vi "HFRR ADV v12.vi"() -> ()   [LabVIEW 2025] (continued)
                frame 88 {
                  n3635 = local write "S 90"(w4921) -> ()
                }
                frame 89 {
                  n3636 = local write "S 91"(w4922) -> ()
                }
                frame 90 {
                  n3637 = local write "S 92"(w4923) -> ()
                }
                frame 91 {
                  n3638 = local write "S 93"(w4924) -> ()
                }
                frame 92 {
                  n3639 = local write "S 94"(w4925) -> ()
                }
                frame 93 {
                  n3640 = local write "S 95"(w4926) -> ()
                }
                frame 94 {
                  n3641 = local write "S 96"(w4927) -> ()
                }
                frame 95 {
                  n3642 = local write "S 97"(w4928) -> ()
                }
                frame 96 {
                  n3643 = local write "S 98"(w4929) -> ()
                }
                frame 97 {
                  n3644 = local write "S 99"(w4930) -> ()
                }
                frame 98 {
                  n3645 = local write "S 100"(w4931) -> ()
                }
                frame 99 {
                  n3646 = local write "S 101"(w4932) -> ()
                }
                frame 100 {
                  n3647 = local write "S 102"(w4933) -> ()
                }
                frame 101 {
                  n3648 = local write "S 103"(w4934) -> ()
                }
                frame 102 {
                  n3649 = local write "S 104"(w4935) -> ()
                }
                frame 103 {
                  n3650 = local write "S 105"(w4936) -> ()
                }
                frame 104 {
                  n3651 = local write "S 106"(w4937) -> ()
                }
                frame 105 {
                }
                frame 106 {
                  n3652 = property on="OK Button 17" class="Bool (strict)"("Boolean Text.Text"=w4938) -> ()  [unwired: 2 in, 2 out]
                }
                frame 107 {
                  n3653 = property on="OK Button 16" class="Bool (strict)"("Boolean Text.Text"=w4939) -> ()  [unwired: 2 in, 2 out]
                }
                frame 108 {
                  n3654 = property on="TITTLE" class="Str"("Caption.Text"=w4940) -> ()  [unwired: 2 in, 2 out]
                }
                frame 109 {
                  "String 30" <- w4941
                }
                frame 110 {
                  n3655 = property on="Test Date" class="Str"("Caption.Text"=w4942) -> ()  [unwired: 2 in, 2 out]
                  "String 31" <- w4942
                }
                frame 111 {
                  n3656 = property on="Sample ID" class="Str"("Caption.Text"=w4943) -> ()  [unwired: 2 in, 2 out]
                  "String 32" <- w4943
                }
                frame 112 {
                  n3657 = property on="Tested by" class="Str"("Caption.Text"=w4944) -> ()  [unwired: 2 in, 2 out]
                  "String 33" <- w4944
                }
                frame 113 {
                  n3658 = property on="System Configured Printers 2" class="Arr (strict)"("Caption.Text"=w4945) -> ()  [unwired: 2 in, 2 out]
                }
                frame 114 {
                  n3659 = property on="Selected Printer" class="Str"("Caption.Text"=w4946) -> ()  [unwired: 2 in, 2 out]
                }
                frame 115 {
                  n3660 = property on="Select Printer 3" class="DigNum (strict)"("Caption.Text"=w4947) -> ()  [unwired: 2 in, 2 out]
                }
                frame 116 {
                  n3661 = property on="Print" class="Bool (strict)"("Boolean Text.Text"=w4948) -> ()  [unwired: 2 in, 2 out]
                }
                frame 117 {
                  "String 41" <- w4949
                }
                frame 118 {
                  n3662 = property on="tested by" class="Str"("Caption.Text"=w4950) -> ()  [unwired: 2 in, 2 out]
                }
                frame 119 {
                }
                frame 120 {
                  n3663 = property on="Export" class="Bool (strict)"("Boolean Text.Text"=w4951) -> ()  [unwired: 2 in, 2 out]
                }
                frame 121 {
                  n3664 = property on="TEMP INTERCEPT:" class="DigNum (strict)"("Caption.Text"=w4952) -> ()  [unwired: 2 in, 2 out]
                }
                frame 122 {
                  n3665 = property on="AIR TEMP INTERCEPT:" class="DigNum (strict)"("Caption.Text"=w4953) -> ()  [unwired: 2 in, 2 out]
                }
                frame 123 {
                  n3666 = property on="Select File Type" class="Enum (strict)"("Caption.Text"=w4954) -> ()  [unwired: 2 in, 2 out]
                }
                frame 124 {
                  n3667 = property on="s.NO" class="Str"("Caption.Text"=w4955) -> ()  [unwired: 2 in, 2 out]
                  "String 45" <- w4955
                }
                frame 125 {
                  n3668 = property on="trip1 8" class="Bool (strict)"("Boolean Text.Text"=w4956) -> ()  [unwired: 2 in, 2 out]
                }
                frame 126, Default {
                }
              }
            }
          }
          frame #1 {
            w4964 = TRUE ("Visible")
            n3669 = local read "S 91"() -> (w4981:string)
            n3670 = local read "S 90"() -> (w4980:string)
            n3671 = local read "S 88"() -> (w4979:string)
            n3672 = property on="Threshold" class="DigNum (strict)"("Caption.Text"=w4981) -> ()  [unwired: 2 in, 2 out]
            n3673 = property on="File Path" class="Path"("Caption.Text"=w4980) -> ()  [unwired: 2 in, 2 out]
            n3674 = property on="SrvM CP" class="Bool (strict)"("Boolean Text.Text"=w4979) -> ()  [unwired: 2 in, 2 out]
            n3675 = local read "S 71"() -> (w4974:string)
            n3676 = local read "S 86"() -> (w4976:string)
            n3677 = local read "S 85"() -> (w4977:string)
            n3678 = local read "S 87"() -> (w4975:string)
            n3679 = local read "S 84"() -> (w4978:string)
            n3680 = local read "S 103"() -> (w4963:string)
            n3681 = local read "S 104"() -> (w4962:string)
            n3682 = property on="ENTER THE NEW PASSWORD" class="Str"("Caption.Text"=w4975) -> ()  [unwired: 2 in, 2 out]
            n3683 = property on="Password" class="Str"("Caption.Text"=w4977) -> ()  [unwired: 2 in, 2 out]
            n3684 = property on="ENTER CURRENT PASSWORD" class="Str"("Caption.Text"=w4976) -> ()  [unwired: 2 in, 2 out]
            n3685 = property on="EDIT" class="Bool (strict)"("Boolean Text.Text"=w4974) -> ()  [unwired: 2 in, 2 out]
            n3686 = property on="SAVE" class="Bool (strict)"("Boolean Text.Text"=w4978) -> ()  [unwired: 2 in, 2 out]
            n3687 = Build Array(w4963, w4962) -> (w4961:string[])
            n3688 = property on="Heater Button" class="Bool (strict)"("Strings [4]"=w4961) -> ()  [unwired: 2 in, 2 out]
            n3689 = property on="CH-HUMIDITY WET" class="DigNum (strict)"("Caption.Size to Text?"=w4964) -> ()  [unwired: 2 in, 2 out]
            n3690 = property on="CH-HUMIDITY DRY" class="DigNum (strict)"("Caption.Size to Text?"=w4964) -> ()  [unwired: 2 in, 2 out]
            n3691 = property on="CH-POWER -" class="DigNum (strict)"("Caption.Size to Text?"=w4964) -> ()  [unwired: 2 in, 2 out]
            n3692 = property on="CH-HEATER" class="DigNum (strict)"("Caption.Size to Text?"=w4964) -> ()  [unwired: 2 in, 2 out]
            n3693 = property on="CH-POWER +" class="DigNum (strict)"("Caption.Size to Text?"=w4964) -> ()  [unwired: 2 in, 2 out]
            n3694 = local read "S 92"() -> (w4973:string)
            n3695 = local read "S 93"() -> (w4972:string)
            n3696 = local read "S 105"() -> (w4959:string)
            n3697 = local read "S 106"() -> (w4958:string)
            n3698 = Build Array(w4973, w4972) -> ()  [unwired: 1 out]
            n3699 = Build Array(w4959, w4958) -> (w4960:string[])
            n3700 = local read "S 95"() -> (w4970:string)
            n3701 = local read "S 94"() -> (w4971:string)
            n3702 = local read "bs"() -> (w4986:string)
            n3703 = local read "as"() -> (w4987:string)
            n3704 = property on="Humidity" class="Bool (strict)"("Strings [4]"=w4960) -> ()  [unwired: 2 in, 2 out]
            n3705 = Concatenate Strings(w4986, "\r", w4987) -> ()  [unwired: 1 out]
            n3706 = property on="STROKE GAIN :" class="DigNum (strict)"("Caption.Text"=w4970) -> ()  [unwired: 2 in, 2 out]
            n3707 = property on="DISPLACEMENT :" class="DigNum (strict)"("Caption.Text"=w4971) -> ()  [unwired: 2 in, 2 out]
            n3708 = property on="Rh After" class="DigNum (strict)"("Caption.Size to Text?"=TRUE ("Caption.Size to Text")) -> ()  [unwired: 2 in, 2 out]
            n3709 = local read "S 48"() -> (w5010:string)
            n3710 = local read "S 50"() -> (w5008:string)
            n3711 = local read "S 51"() -> (w5007:string)
            n3712 = local read "S 49"() -> (w5009:string)
            n3713 = local read "S 52"() -> (w5006:string)
            n3714 = local read "as"() -> (w4991:string)
            n3715 = local read "bs"() -> (w4992:string)
            n3716 = local read "S 56"() -> (w5005:string)
            n3717 = local read "S 57"() -> (w5004:string)
            n3718 = local read "S 58"() -> (w5003:string)
            n3719 = local read "S 59"() -> (w5002:string)
            n3720 = property on="OPEN" class="Bool (strict)"("Boolean Text.Text"=w5006) -> ()  [unwired: 2 in, 2 out]
            n3721 = property on="OPEN 1" class="Bool (strict)"("Boolean Text.Text"=w5010) -> ()  [unwired: 2 in, 2 out]
            n3722 = property on="OPEN 2" class="Bool (strict)"("Boolean Text.Text"=w5009) -> ()  [unwired: 2 in, 2 out]
            n3723 = property on="OPEN 3" class="Bool (strict)"("Boolean Text.Text"=w5008) -> ()  [unwired: 2 in, 2 out]
            n3724 = property on="OPEN 4" class="Bool (strict)"("Boolean Text.Text"=w5007) -> ()  [unwired: 2 in, 2 out]
            n3725 = Concatenate Strings(w4992, "\r", w4991) -> ()  [unwired: 1 out]
            n3726 = local read "S 102"() -> (w4965:string)
            n3727 = property on="КОФ1" class="DigNum (strict)"("Caption.Text"=w5005) -> ()  [unwired: 2 in, 2 out]
            n3728 = local read "S 98"() -> (w4969:string)
            n3729 = local read "S 99"() -> (w4968:string)
            n3730 = local read "S 100"() -> (w4967:string)
            n3731 = local read "S 101"() -> (w4966:string)
            n3732 = property on="КОФ2" class="DigNum (strict)"("Caption.Text"=w5004) -> ()  [unwired: 2 in, 2 out]
            n3733 = property on="КОФ3" class="DigNum (strict)"("Caption.Text"=w5003) -> ()  [unwired: 2 in, 2 out]
            n3734 = property on="КОФ4" class="DigNum (strict)"("Caption.Text"=w5002) -> ()  [unwired: 2 in, 2 out]
            n3735 = local read "bs"() -> (w4990:string)
            n3736 = local read "as"() -> (w4989:string)
            n3737 = property on="CH-POWER +" class="DigNum (strict)"("Caption.Text"=w4969) -> ()  [unwired: 2 in, 2 out]
            n3738 = property on="CH-POWER -" class="DigNum (strict)"("Caption.Text"=w4968) -> ()  [unwired: 2 in, 2 out]
            n3739 = property on="CH-HEATER" class="DigNum (strict)"("Caption.Text"=w4967) -> ()  [unwired: 2 in, 2 out]
            n3740 = property on="CH-HUMIDITY DRY" class="DigNum (strict)"("Caption.Text"=w4966) -> ()  [unwired: 2 in, 2 out]
            n3741 = property on="CH-HUMIDITY WET" class="DigNum (strict)"("Caption.Text"=w4965) -> ()  [unwired: 2 in, 2 out]
            n3742 = local read "S 60"() -> (w5001:string)
            n3743 = local read "S 54"() -> (w5011:string)
            n3744 = Concatenate Strings(w4990, "\r", w4989) -> ()  [unwired: 1 out]
            n3745 = Concatenate Strings(w5011, w5001) -> ()  [unwired: 1 out]
            n3746 = local read "S 77"() -> (→"String 43":string)
            n3747 = local read "S 76"() -> (w4984:string)
            n3748 = local read "S 78"() -> (w4983:string)
            n3749 = local read "S 71"() -> (w4995:string)
            n3750 = local read "S 66"() -> (w5000:string)
            n3751 = local read "S 67"() -> (w4999:string)
            n3752 = local read "S 68"() -> (w4998:string)
            n3753 = local read "S 69"() -> (w4997:string)
            n3754 = local read "S 70"() -> (w4996:string)
            n3755 = property on="AIR TEMP" class="DigNum (strict)"("Caption.Text"=w4983) -> ()  [unwired: 2 in, 2 out]
            n3756 = property on="Set Strk" class="DigNum (strict)"("Caption.Text"=w4984) -> ()  [unwired: 2 in, 2 out]
            n3757 = property on="FRIC. FORCE :" class="DigNum (strict)"("Caption.Text"=w5000) -> ()  [unwired: 2 in, 2 out]
            n3758 = property on="TEMPERATURE :" class="DigNum (strict)"("Caption.Text"=w4999) -> ()  [unwired: 2 in, 2 out]
            n3759 = property on="SPEED OUT:" class="DigNum (strict)"("Caption.Text"=w4998) -> ()  [unwired: 2 in, 2 out]
            n3760 = property on="AIR TEMPERATURE :" class="DigNum (strict)"("Caption.Text"=w4997) -> ()  [unwired: 2 in, 2 out]
            n3761 = property on="HUMIDITY:" class="DigNum (strict)"("Caption.Text"=w4996) -> ()  [unwired: 2 in, 2 out]
            n3762 = property on="EDIT" class="Bool (strict)"("Boolean Text.Text"=w4995) -> ()  [unwired: 2 in, 2 out]
            n3763 = local read "S 79"() -> (w4982:string)
            n3764 = property on="Stroke" class="DigNum (strict)"("Caption.Text"=w4982) -> ()  [unwired: 2 in, 2 out]
          }
          frame #2 {
          }
        }
        n3765 = local write "Lan flag"(10.0 ("Lan flag")) -> ()
      }
      frame Enabled {
      }
    }
    n3766 = Wait (ms)(milliseconds to wait=u32 2000) -> ()  [unwired: 1 out]
    n3767 = local read "Quit"() -> (w4784:bool)
  }
  n3768 = disable-structure shown="Disabled" {
    frame Disabled {
      n3769 = while {
        tunnel: [w5013] -> _
        i -> [w5013]
        stop <- w5012 continue-if-true
        n3770 = Wait (ms)(milliseconds to wait=u32 50) -> ()  [unwired: 1 out]
        n3771 = stacked-sequence {
          frame #0 {
            # "Controls Text color"
            # "Controls BG color"
            n3772 = property on="FILE" class="Str"("Text.Text Colors:Text Color"="SC  Text") -> ()  [unwired: 2 in, 2 out]
            n3773 = property on="Fuel Discription :" class="Str"("Text.Text Colors:Text Color"="SC  Text") -> ()  [unwired: 2 in, 2 out]
            n3774 = property on="tested by" class="Str"("Text.Text Colors:Text Color"="SC  Text") -> ()  [unwired: 2 in, 2 out]
            n3775 = property on="Remarks :" class="Str"("Text.Text Colors:Text Color"="SC  Text") -> ()  [unwired: 2 in, 2 out]
            n3776 = property class="DigNum (strict)"("Numeric Text.Text Colors:BG Color"="NC BG") -> ()  [unwired: 2 in, 2 out]
            n3777 = property class="DigNum (strict)"("Numeric Text.Text Colors:BG Color"="NC BG") -> ()  [unwired: 2 in, 2 out]
            n3778 = property class="DigNum (strict)"("Numeric Text.Text Colors:BG Color"="NC BG") -> ()  [unwired: 2 in, 2 out]
            n3779 = property class="DigNum (strict)"("Numeric Text.Text Colors:BG Color"="NC BG") -> ()  [unwired: 2 in, 2 out]
            n3780 = property class="DigNum (strict)"("Numeric Text.Text Colors:BG Color"="NC BG") -> ()  [unwired: 2 in, 2 out]
            n3781 = property class="DigNum (strict)"("Numeric Text.Text Colors:BG Color"="NC BG") -> ()  [unwired: 2 in, 2 out]
            n3782 = property class="DigNum (strict)"("Numeric Text.Text Colors:BG Color"="NC BG") -> ()  [unwired: 2 in, 2 out]
            n3783 = property class="DigNum (strict)"("Numeric Text.Text Colors:BG Color"="NC BG") -> ()  [unwired: 2 in, 2 out]
            n3784 = property class="DigNum (strict)"("Numeric Text.Text Colors:BG Color"="NC BG") -> ()  [unwired: 2 in, 2 out]
            n3785 = property class="DigNum (strict)"("Numeric Text.Text Colors:BG Color"="NC BG") -> ()  [unwired: 2 in, 2 out]
            n3786 = property class="DigNum (strict)"("Numeric Text.Text Colors:BG Color"="NC BG") -> ()  [unwired: 2 in, 2 out]
            n3787 = property class="DigNum (strict)"("Numeric Text.Text Colors:BG Color"="NC BG") -> ()  [unwired: 2 in, 2 out]
            n3788 = property on="FILE" class="Str"("Text.Text Colors:BG Color"="SC BG 3") -> ()  [unwired: 2 in, 2 out]
            n3789 = property on="Fuel Discription :" class="Str"("Text.Text Colors:BG Color"="SC BG 3") -> ()  [unwired: 2 in, 2 out]
            n3790 = property on="tested by" class="Str"("Text.Text Colors:BG Color"="SC BG 3") -> ()  [unwired: 2 in, 2 out]
            n3791 = property on="Remarks :" class="Str"("Text.Text Colors:BG Color"="SC BG 3") -> ()  [unwired: 2 in, 2 out]
            n3792 = property class="DigNum (strict)"("Numeric Text.Text Colors:Text Color"="NC Text") -> ()  [unwired: 2 in, 2 out]
            n3793 = property class="DigNum (strict)"("Numeric Text.Text Colors:Text Color"="NC Text") -> ()  [unwired: 2 in, 2 out]
            n3794 = property class="DigNum (strict)"("Numeric Text.Text Colors:Text Color"="NC Text") -> ()  [unwired: 2 in, 2 out]
            n3795 = property class="DigNum (strict)"("Numeric Text.Text Colors:Text Color"="NC Text") -> ()  [unwired: 2 in, 2 out]
            n3796 = property class="DigNum (strict)"("Numeric Text.Text Colors:Text Color"="NC Text") -> ()  [unwired: 2 in, 2 out]
            n3797 = property class="DigNum (strict)"("Numeric Text.Text Colors:Text Color"="NC Text") -> ()  [unwired: 2 in, 2 out]
            n3798 = property class="DigNum (strict)"("Numeric Text.Text Colors:Text Color"="NC Text") -> ()  [unwired: 2 in, 2 out]
            n3799 = property class="DigNum (strict)"("Numeric Text.Text Colors:Text Color"="NC Text") -> ()  [unwired: 2 in, 2 out]
            n3800 = property class="DigNum (strict)"("Numeric Text.Text Colors:Text Color"="NC Text") -> ()  [unwired: 2 in, 2 out]
            n3801 = property class="DigNum (strict)"("Numeric Text.Text Colors:Text Color"="NC Text") -> ()  [unwired: 2 in, 2 out]
            n3802 = property class="DigNum (strict)"("Numeric Text.Text Colors:Text Color"="NC Text") -> ()  [unwired: 2 in, 2 out]
            n3803 = property class="DigNum (strict)"("Numeric Text.Text Colors:Text Color"="NC Text") -> ()  [unwired: 2 in, 2 out]
            n3804 = property class="DigNum (strict)"("Numeric Text.Text Colors:Text Color"="NI Text  2") -> ()  [unwired: 2 in, 2 out]
            n3805 = property class="DigNum (strict)"("Numeric Text.Text Colors:Text Color"="NI Text  2") -> ()  [unwired: 2 in, 2 out]
            n3806 = property class="DigNum (strict)"("Numeric Text.Text Colors:Text Color"="NI Text  2") -> ()  [unwired: 2 in, 2 out]
            n3807 = property class="DigNum (strict)"("Numeric Text.Text Colors:Text Color"="NI Text  2") -> ()  [unwired: 2 in, 2 out]
            n3808 = property class="DigNum (strict)"("Numeric Text.Text Colors:Text Color"="NI Text  2") -> ()  [unwired: 2 in, 2 out]
            n3809 = property class="DigNum (strict)"("Numeric Text.Text Colors:Text Color"="NI Text  2") -> ()  [unwired: 2 in, 2 out]
            n3810 = property class="DigNum (strict)"("Numeric Text.Text Colors:Text Color"="NI Text  2") -> ()  [unwired: 2 in, 2 out]
            n3811 = property class="DigNum (strict)"("Numeric Text.Text Colors:Text Color"="NI Text  2") -> ()  [unwired: 2 in, 2 out]
            n3812 = property class="DigNum (strict)"("Numeric Text.Text Colors:Text Color"="NI Text  2") -> ()  [unwired: 2 in, 2 out]
            n3813 = property class="DigNum (strict)"("Numeric Text.Text Colors:Text Color"="NI Text  2") -> ()  [unwired: 2 in, 2 out]
            n3814 = property class="DigNum (strict)"("Numeric Text.Text Colors:Text Color"="NI Text  2") -> ()  [unwired: 2 in, 2 out]
            n3815 = property class="DigNum (strict)"("Numeric Text.Text Colors:Text Color"="NI Text  2") -> ()  [unwired: 2 in, 2 out]
            n3816 = property class="DigNum (strict)"("Numeric Text.Text Colors:Text Color"="NI Text  2") -> ()  [unwired: 2 in, 2 out]
            n3817 = property class="DigNum (strict)"("Numeric Text.Text Colors:Text Color"="NI Text  2") -> ()  [unwired: 2 in, 2 out]
            n3818 = property class="DigNum (strict)"("Numeric Text.Text Colors:Text Color"="NI Text  2") -> ()  [unwired: 2 in, 2 out]
            n3819 = property class="DigNum (strict)"("Numeric Text.Text Colors:Text Color"="NI Text  2") -> ()  [unwired: 2 in, 2 out]
            n3820 = property on="Coefficient Of Friction" class="XYGraph (strict)"("Plot Area:Colors:FG Color"="GFG  2", "Plot Area:Colors:BG Color"="GBG   2") -> ()  [unwired: 2 in, 2 out]
            n3821 = property on="Humidity ( %RH )" class="XYGraph (strict)"("Plot Area:Colors:FG Color"="GFG  2", "Plot Area:Colors:BG Color"="GBG   2") -> ()  [unwired: 2 in, 2 out]
            n3822 = property on="Air Temperature  ( °C )" class="XYGraph (strict)"("Plot Area:Colors:FG Color"="GFG  2", "Plot Area:Colors:BG Color"="GBG   2") -> ()  [unwired: 2 in, 2 out]
            n3823 = property on="Sample Temperature ( °C )" class="XYGraph (strict)"("Plot Area:Colors:FG Color"="GFG  2", "Plot Area:Colors:BG Color"="GBG   2") -> ()  [unwired: 2 in, 2 out]
            n3824 = property class="DigNum (strict)"("Numeric Text.Text Colors:BG Color"="NI BG 2") -> ()  [unwired: 2 in, 2 out]
            n3825 = property class="DigNum (strict)"("Numeric Text.Text Colors:BG Color"="NI BG 2") -> ()  [unwired: 2 in, 2 out]
            n3826 = property class="DigNum (strict)"("Numeric Text.Text Colors:BG Color"="NI BG 2") -> ()  [unwired: 2 in, 2 out]
            n3827 = property class="DigNum (strict)"("Numeric Text.Text Colors:BG Color"="NI BG 2") -> ()  [unwired: 2 in, 2 out]
            n3828 = property class="DigNum (strict)"("Numeric Text.Text Colors:BG Color"="NI BG 2") -> ()  [unwired: 2 in, 2 out]
            n3829 = property class="DigNum (strict)"("Numeric Text.Text Colors:BG Color"="NI BG 2") -> ()  [unwired: 2 in, 2 out]
            n3830 = property class="DigNum (strict)"("Numeric Text.Text Colors:BG Color"="NI BG 2") -> ()  [unwired: 2 in, 2 out]
            n3831 = property class="DigNum (strict)"("Numeric Text.Text Colors:BG Color"="NI BG 2") -> ()  [unwired: 2 in, 2 out]
            n3832 = property class="DigNum (strict)"("Numeric Text.Text Colors:BG Color"="NI BG 2") -> ()  [unwired: 2 in, 2 out]
            n3833 = property class="DigNum (strict)"("Numeric Text.Text Colors:BG Color"="NI BG 2") -> ()  [unwired: 2 in, 2 out]
            n3834 = property class="DigNum (strict)"("Numeric Text.Text Colors:BG Color"="NI BG 2") -> ()  [unwired: 2 in, 2 out]
            n3835 = property class="DigNum (strict)"("Numeric Text.Text Colors:BG Color"="NI BG 2") -> ()  [unwired: 2 in, 2 out]
            n3836 = property class="DigNum (strict)"("Numeric Text.Text Colors:BG Color"="NI BG 2") -> ()  [unwired: 2 in, 2 out]
            n3837 = property class="DigNum (strict)"("Numeric Text.Text Colors:BG Color"="NI BG 2") -> ()  [unwired: 2 in, 2 out]
            n3838 = property class="DigNum (strict)"("Numeric Text.Text Colors:BG Color"="NI BG 2") -> ()  [unwired: 2 in, 2 out]
            n3839 = property class="DigNum (strict)"("Numeric Text.Text Colors:BG Color"="NI BG 2") -> ()  [unwired: 2 in, 2 out]
            n3840 = property class="Bool"("Colors [4]"="Boolean BC T & BG") -> ()  [unwired: 2 in, 2 out]
            n3841 = property on="Save & Continue" class="Bool (strict)"("Colors [4]"="Boolean BC T & BG") -> ()  [unwired: 2 in, 2 out]
            n3842 = property on="Heater Button" class="Bool (strict)"("Colors [4]"="Boolean BC T & BG") -> ()  [unwired: 2 in, 2 out]
            n3843 = property class="Bool"("Colors [4]"="Boolean BC T & BG") -> ()  [unwired: 2 in, 2 out]
            n3844 = property on="Humidity" class="Bool (strict)"("Colors [4]"="Boolean BC T & BG") -> ()  [unwired: 2 in, 2 out]
            n3845 = property class="Bool (strict)"("Colors [4]"="Boolean BC T & BG") -> ()  [unwired: 2 in, 2 out]
            n3846 = property on="RUN" class="Bool (strict)"("Colors [4]"="Boolean BC T & BG") -> ()  [unwired: 2 in, 2 out]
            n3847 = property on="trip1 8" class="Bool (strict)"("Colors [4]"="Boolean BC T & BG") -> ()  [unwired: 2 in, 2 out]
            n3848 = property class="Bool"("Colors [4]"="Boolean BC T & BG") -> ()  [unwired: 2 in, 2 out]
            n3849 = property class="Bool (strict)"("Colors [4]"="Boolean BC T & BG") -> ()  [unwired: 2 in, 2 out]
            n3850 = property on="OPEN 1" class="Bool (strict)"("Colors [4]"="Boolean BC T & BG 2") -> ()  [unwired: 2 in, 2 out]
            n3851 = property on="OPEN 2" class="Bool (strict)"("Colors [4]"="Boolean BC T & BG 2") -> ()  [unwired: 2 in, 2 out]
            n3852 = property on="OPEN 3" class="Bool (strict)"("Colors [4]"="Boolean BC T & BG 2") -> ()  [unwired: 2 in, 2 out]
            n3853 = property on="OPEN 4" class="Bool (strict)"("Colors [4]"="Boolean BC T & BG 2") -> ()  [unwired: 2 in, 2 out]
            n3854 = property on="OPEN" class="Bool (strict)"("Colors [4]"="Boolean BC T & BG 2") -> ()  [unwired: 2 in, 2 out]
            n3855 = property on="rstv2" class="Bool"("Colors [4]"="Boolean BC T & BG 2") -> ()  [unwired: 2 in, 2 out]
            n3856 = property on="RST CP" class="Bool"("Colors [4]"="Boolean BC T & BG 2") -> ()  [unwired: 2 in, 2 out]
            n3857 = property on="RSTV1 3" class="Bool"("Colors [4]"="Boolean BC T & BG 2") -> ()  [unwired: 2 in, 2 out]
            n3858 = property on="RSTV1 2" class="Bool"("Colors [4]"="Boolean BC T & BG 2") -> ()  [unwired: 2 in, 2 out]
          }
          frame #1 {
          }
        }
        n3859 = local read "Quit"() -> (w5012:bool)
      }
    }
    frame Enabled {
    }
  }
  n3860 = while {
    shift-right: [w5030] -> _
    shift-left: _ -> [w5031]
    shift-right: [w5028] -> _
    shift-left: T17 {"Read Heave and Surge"="", "Bytes at Heave Port"=0.0, "Heave and Surge COM Port:"="COM9", "Com Port 2"="COM7", "Residual Due"="", "Heave COM Status 2"=TRUE, "Heave COM Status"=TRUE, "Port 2"=TRUE, "Sway PPR"=6400.0, "Surge PPR"=6400.0, "Heave PPR"=6400.0, "Sway Pitch"=2.0, "Surge Pitch"=3.0, "Heave Pitch"=4.0, "Sway Pulses/mm"=320.0, "Surge Pulses/mm"=1600.0, "Heave Pulses/mm"=1600.0, "inner loop"=0.0, "Read Heave and Surge 2"="", "String 36"="", "Write S"=FALSE, "WriteCC1"=[""], "Heave COM Loop"=0, "LastCom"="", "EXIT"=FALSE, "Error Heave"={"status"=TRUE, "code"=-1073807343, "source"=""}} -> [w5027]
    shift-right: [w5025] -> _
    shift-left: enum16{"init", "MAIN", "Panel Close"}."init" -> [w5026]
    stop <- w5029 stop-if-true
    n3861 = case shown="\"init\"" w5026 {
      tunnel: w5031 -> [w5045 w5060 w5130 w5132]
      tunnel: [w5039 w5078 w5130 w5132] -> w5030
      tunnel: [_ _ TRUE _] -> w5029
      tunnel: [w5035 w5075 w5128 w5131] -> w5028
      tunnel: w5027 -> [w5042 w5059 w5128 w5131]
      tunnel: [enum16{"init", "MAIN", "Panel Close"}."MAIN" w5053 _ _] -> w5025
      frame "init" {
        n3862 = Bundle By Name(cluster=w5042, "Heave and Surge COM Port:"="C3 :") -> (w5041:T17)
        n3863 = call "Instrument fgv.vi"("Enum"=T27."INIT", "error in (no error) 2"=w5045, "INPUT"=w5041) -> ("error"=w5043:errorcluster, "output"=w5038:T17)  [unwired: 6 in, 1 out]
        n3864 = case shown="No Error" w5043 {
          selector: w5043 -> [w5047 _]
          tunnel: [w5047 w5051] -> w5039
          tunnel: w5038 -> [w5046 w5049]
          tunnel: [w5046 w5048] -> w5036
          frame No Error {
          }
          frame Error {
            n3865 = call "Instrument fgv.vi"("Enum"=T27."ERROR INIT", "INPUT"=w5049) -> ("error"=w5052:errorcluster, "output"=w5048:T17)  [unwired: 7 in, 1 out]
            n3866 = call <vilib>:"Clear Errors.vi"("error in (no error)"=w5052) -> ("error out"=w5051:errorcluster)  [unwired: 5 in, 1 out]
          }
        }
        n3867 = local read "LastCom"() -> (w5034:string)
        n3868 = Unbundle By Name(w5036) -> ("Heave COM Status 2"=→"COM Status" →"Instrument Status":bool, "Error Heave"=→"Error":errorcluster)  [unwired: 1 out]
        n3869 = Bundle By Name(cluster=w5036, "LastCom"=w5034) -> (w5035:T17)
      }
      frame "MAIN" {
        n3870 = Unbundle By Name(w5059) -> ("Com Port 2"=w5080:refnum<visa-resource-name>)
        n3871 = local write "Com Port 4"(w5080) -> ()
        n3872 = local read "C3 :"() -> (w5057:refnum<visa-resource-name>)
        n3873 = Divide(x="Heave PPR", y="Heave Pitch") -> (x/y=→"Heave Pulses/mm":dbl)
        n3874 = Bundle By Name(cluster=w5059, "Heave and Surge COM Port:"=w5057) -> (w5058:T17)
        n3875 = Equal?(x=w5080, y=w5057) -> (x = y?=w5079:bool)
        n3876 = Divide(x="Sway PPR", y="Sway Pitch") -> (x/y=→"Sway Pulses/mm":dbl)
        n3877 = case shown="False" w5079 {
          tunnel: [w5084 w5101] -> w5078
          tunnel: w5060 -> [w5085 w5107]
          tunnel: w5058 -> [w5083 w5105]
          tunnel: [w5082 w5100] -> w5075
          frame False {
            n3878 = call <vilib>:"Clear Errors.vi"("error in (no error)"=w5085) -> ("error out"=w5081:errorcluster)  [unwired: 5 in, 1 out]
            n3879 = call "Instrument fgv.vi"("Enum"=T27."ERROR INIT", "error in (no error) 2"=w5081, "INPUT"=w5083) -> ("error"=w5087:errorcluster, "output"=w5082:T17)  [unwired: 6 in, 1 out]
            n3880 = call <vilib>:"Clear Errors.vi"("error in (no error)"=w5087) -> ("error out"=w5084:errorcluster)  [unwired: 5 in, 1 out]
          }
          frame True {
            n3881 = call "Instrument fgv.vi"("Enum"=T27."READ", "error in (no error) 2"=w5107, "INPUT"=w5105) -> ("error"=w5106:errorcluster, "output"=w5097:T17)  [unwired: 6 in, 1 out]
            n3882 = Bundle By Name(cluster=w5097, "String 36"="String 11") -> (w5096:T17)
            n3883 = case shown="True" "Write S" {
              selector: "Write S" -> [_ w5127]
              tunnel: w5106 -> [w5120 w5126]
              tunnel: [w5120 w5125] -> w5093
              tunnel: w5096 -> [w5119 w5122]
              tunnel: [w5119 w5121] -> w5092
              frame False {
              }
              frame True {
                n3884 = Not(x=w5127) -> (.not. x?=w5123:bool)
                n3885 = local write "Write S"(w5123) -> ()
                n3886 = call "Instrument fgv.vi"("Enum"=T27."MANUAL WRITE", "error in (no error) 2"=w5126, "INPUT"=w5122) -> ("error"=w5125:errorcluster, "output"=w5121:T17)  [unwired: 6 in, 1 out]
              }
            }
            n3887 = Array Size(array="WriteHumidity") -> (size(s)=w5090:i32)
            n3888 = Greater Than 0?(x=w5090) -> (x > 0?=w5088:bool)
            n3889 = call "Instrument fgv.vi"("Enum"=T27."WRITE", "error in (no error) 2"=w5093, "WriteCC1"="WriteHumidity", "INPUT"=w5092) -> ("error"=w5103:errorcluster, "WriteCC1 2"=w5091:string[], "output"=w5102:T17)  [unwired: 5 in]
            n3890 = case shown="True" w5088 {
              tunnel: w5091 -> [_ w5109]
              frame False {
              }
              frame True {
                n3891 = local write "WriteHumidity"(w5109) -> ()
              }
            }
            n3892 = case shown="Error" w5103 {
              selector: w5103 -> [w5110 w5113]
              tunnel: w5102 -> [w5111 w5118]
              tunnel: [w5111 w5117] -> w5100
              tunnel: [w5110 w5115] -> w5101
              frame No Error {
              }
              frame Error {
                n3893 = call <vilib>:"Clear Errors.vi"("error in (no error)"=w5113) -> ("error out"=w5112:errorcluster)  [unwired: 5 in, 1 out]
                n3894 = call "Instrument fgv.vi"("Enum"=T27."ERROR INIT", "error in (no error) 2"=w5112, "INPUT"=w5118) -> ("error"=w5116:errorcluster, "output"=w5117:T17)  [unwired: 6 in, 1 out]
                n3895 = call <vilib>:"Clear Errors.vi"("error in (no error)"=w5116) -> ("error out"=w5115:errorcluster)  [unwired: 5 in, 1 out]
              }
            }
            n3896 = Unbundle By Name(w5100) -> ("LastCom"=→"LastCom":string, "Read Heave and Surge"=→"Read Humidity":string)
          }
        }
        n3897 = Divide(x="Surge PPR", y="Surge Pitch") -> (x/y=→"Surge Pulses/mm":dbl)
        n3898 = Unbundle By Name(w5075) -> ("Heave COM Status 2"=w5077:bool, "Heave COM Status"=w5076:bool, "Error Heave"=w5073:errorcluster, "Bytes at Heave Port"=→"Bytes at Humidity Port":dbl)
        n3899 = Unbundle By Name(w5073) -> ("status"=→"Humidity Port":bool)
        n3900 = Not(x=w5076) -> (.not. x?=w5061:bool)
        n3901 = local write "Error"(w5073) -> ()
        n3902 = Not(x=w5077) -> (.not. x?=w5062:bool)
        n3903 = local write "Instrument Status"(w5061) -> ()
        n3904 = local write "COM Status"(w5062) -> ()
        n3905 = local read "Quit"() -> (w5054:bool)
        n3906 = Select(t=enum16{"init", "MAIN", "Panel Close"}."Panel Close", s=w5054, f=enum16{"init", "MAIN", "Panel Close"}."MAIN") -> (s? t:f=w5053:enum16{"init", "MAIN", "Panel Close"})
      }
      frame "Panel Close" {
      }
      frame Default {
      }
    }
  }
  n3907 = while {
    stop <- w5158 stop-if-true
    n3908 = local read "Read Humidity"() -> (w5139:string)
    n3909 = call <vilib>:"High Resolution Polling Wait.vi"("seconds to wait"=0.1) -> ()  [unwired: 10 in, 1 out]
    n3910 = Spreadsheet String To Array(delimiter (Tab)=",", format string="", spreadsheet string=w5139, array type (2D Dbl)=string[] []) -> (array=w5153:string[])
    n3911 = for {
      tunnel: w5153 -> [w5163] mode=indexing
      tunnel: string[] ["STATE;", "SET;", "RH;", "T;", "AMB_RH;", "AMB_T;", "PUMP;", "FAN_IN;", "FAN_OUT;", "DEHUM;", "CURRENT;", "STALL;"] -> [w5162] mode=indexing
      tunnel: [w5161] -> w5152 mode=indexing
      n3912 = Match Pattern(string=w5163, regular expression=w5162) -> (after substring=w5161:string)  [unwired: 1 in, 3 out]
    }
    n3913 = Index Array(array=w5152) -> (element #1=→"STATE :":string, element #2=→"SET :":string, element #3=w5141:string, element #4=→"T :":string, element #5=w5138:string, element #6=→"AMB_T :":string, element #7=→"PUMP :":string, element #8=→"FAN_IN :":string, element #9=→"FAN_OUT :":string, element #10=→"DEHUM :":string, element #11=→"CURRENT :":string, element #12=→"STALL :":string)  [unwired: 12 in]
    "RH :" <- w5141
    "AMB_RH :" <- w5138
    n3914 = Fract/Exp String To Number(string=w5141) -> (number=w5133:dbl)  [unwired: 3 in, 1 out]
    n3915 = Fract/Exp String To Number(string=w5138) -> (number=w5137:dbl)  [unwired: 3 in, 1 out]
    n3916 = local write "Ambient Humidity :"(w5137) -> ()
    n3917 = Equal?(x=w5133, y=0.0) -> (x = y?=w5135:bool)
    n3918 = case shown="True" w5135 {
      tunnel: [w5159 w5160] -> w5134
      tunnel: w5133 -> [w5159 _]
      frame False {
        (unwired) 0.0
        "Humidity temp" <- w5159
      }
      frame True {
        n3919 = local read "Humidity temp"() -> (w5160:dbl)
      }
    }
    "RH Numeric:" <- w5134
    n3920 = local read "Quit"() -> (w5158:bool)
  }
  n3921 = disable-structure shown="Disabled" {
    frame Disabled {
      n3922 = while {
        tunnel: [w5397] -> _
        i -> [w5397]
        stop <- w5394 stop-if-true
        n3923 = local read "powstat"() -> (w5395:bool)
        n3924 = case shown="True" w5395 {
          frame False {
          }
          frame True {
            n3925 = local read "RUN"() -> (w5398:bool)
            n3926 = case shown="True" w5398 {
              frame False {
                w5428 = 65.0 ("y")
                n3927 = local read "Set Hz"() -> (w5456:dbl)
                n3928 = local read "NORMAL LOAD"() -> (w5457:dbl)
                n3929 = Multiply(x=w5456, y=60.0) -> (x*y=w5463:dbl)
                n3930 = Multiply(x=1.2 ("y"), y=0.949) -> (x*y=w5432:dbl)
                n3931 = Multiply(x=1.2 ("y"), y=0.8166) -> (x*y=w5436:dbl)
                n3932 = Multiply(x=1.2 ("y"), y=0.851) -> (x*y=w5431:dbl)
                n3933 = local read "FF 2"() -> (w5455:dbl)
                n3934 = Absolute Value(x=w5463) -> (abs(x)=w5461:dbl)
                n3935 = local read "Stroke"() -> (w5430:dbl)
                n3936 = Less?(x=w5430, y=w5436) -> (x < y?=w5433:bool)
                n3937 = In Range and Coerce(upper limit=w5432, x=w5430, lower limit=w5431) -> (In Range?=w5434:bool)  [unwired: 1 out]
                n3938 = case shown="13.." w5455 {
                  tunnel: [1 2 3] -> w5453
                  frame 0..10, Default {
                    # "Normal"
                  }
                  frame 11, 12 {
                  }
                  frame 13.. {
                  }
                }
                "FF STATE" <- w5453
                n3939 = local read "TEMP"() -> (w5416:dbl)
                n3940 = case shown="3601.." w5461 {
                  tunnel: [1 2 3] -> w5459
                  frame 0..3000, Default {
                    # "Normal"
                  }
                  frame 3001..3600 {
                  }
                  frame 3601.. {
                  }
                }
                n3941 = case shown="11.." w5457 {
                  tunnel: [1 3] -> w5458
                  frame 1..10, Default {
                  }
                  frame 11.. {
                  }
                }
                "NL STATE" <- w5458
                n3942 = Multiply(x=1.2 ("y"), y=0.95) -> (x*y=w5446:dbl)
                n3943 = Multiply(x=w5428, y=0.954) -> (x*y=w5420:dbl)
                n3944 = Or(x=w5433, y=w5434) -> (x .or. y?=w5435:bool)
                n3945 = Greater Or Equal?(x=w5430, y=w5446) -> (x >= y?=w5443:bool)
                n3946 = Multiply(x=w5428, y=0.99) -> (x*y=w5417:dbl)
                n3947 = Greater Or Equal?(x=w5416, y=w5417) -> (x >= y?=w5422:bool)
                n3948 = Greater Or Equal?(x=w5416, y=w5420) -> (x >= y?=w5419:bool)
                n3949 = case shown="0, 1, Default" w5430 {
                  tunnel: [1 3] -> w5447
                  frame 0, 1, Default {
                  }
                  frame 2.. {
                  }
                }
                n3950 = case shown="True" w5443 {
                  tunnel: [1 3] -> w5448
                  frame False {
                  }
                  frame True {
                  }
                }
                n3951 = case shown="True" w5435 {
                  tunnel: [1 2] -> w5449
                  frame False {
                  }
                  frame True {
                  }
                }
                n3952 = case shown="..0" w5416 {
                  tunnel: [2 3 3 1] -> w5423
                  frame 61, 62 {
                  }
                  frame 63.. {
                  }
                  frame ..0 {
                  }
                  frame 10..60, Default {
                  }
                }
                n3953 = case shown="True" w5422 {
                  tunnel: [1 3] -> w5424
                  frame False {
                  }
                  frame True {
                  }
                }
                n3954 = Number To Decimal String(number=w5459) -> (decimal integer string=w5460:string)  [unwired: 1 in]
                n3955 = case shown="True" w5419 {
                  tunnel: [1 2] -> w5425
                  frame False {
                  }
                  frame True {
                  }
                }
                n3956 = Number To Decimal String(number=1) -> (decimal integer string=→"Air temp":string)  [unwired: 1 in]
                n3957 = Number To Decimal String(number=w5453) -> (decimal integer string=→"ff_st":string)  [unwired: 1 in]
                n3958 = local write "sp_st"(w5460) -> ()
                n3959 = Number To Decimal String(number=w5458) -> (decimal integer string=→"nl_st":string)  [unwired: 1 in]
                n3960 = Build Array(w5423, w5424, w5425) -> (w5426:i32[])
                n3961 = Build Array(w5447, w5448, w5449) -> (w5450:i32[])
                n3962 = Array Max & Min(array=w5426) -> (max value=w5427:i32)  [unwired: 3 out]
                n3963 = Array Max & Min(array=w5450) -> (max value=w5451:i32)  [unwired: 3 out]
                n3964 = Number To Decimal String(number=w5427) -> (decimal integer string=w5415:string)  [unwired: 1 in]
                n3965 = Number To Decimal String(number=w5451) -> (decimal integer string=→"Stroke Ln 2":string)  [unwired: 1 in]
                n3966 = local write "temp_st"(w5415) -> ()
              }
              frame True {
                w5513 = 65.0 ("y")
                # "Healthy -1\nWarning -2\nError -3"
                n3967 = local read "TEMP"() -> (w5524:dbl)
                n3968 = local read "NORMAL LOAD"() -> (w5528:dbl)
                n3969 = local read "Set Hz"() -> (w5526:dbl)
                n3970 = Multiply(x=1.2 ("y"), y=0.949) -> (x*y=w5508:dbl)
                n3971 = Multiply(x=1.2 ("y"), y=0.8166) -> (x*y=w5504:dbl)
                n3972 = Multiply(x=1.2 ("y"), y=0.851) -> (x*y=w5509:dbl)
                n3973 = Multiply(x=w5513, y=0.954) -> (x*y=w5520:dbl)
                n3974 = Multiply(x=w5513, y=0.99) -> (x*y=w5523:dbl)
                n3975 = Greater Or Equal?(x=w5524, y=w5523) -> (x >= y?=w5518:bool)
                n3976 = Multiply(x=w5526, y=60.0) -> (x*y=w5532:dbl)
                n3977 = Greater Or Equal?(x=w5524, y=w5520) -> (x >= y?=w5521:bool)
                n3978 = local read "FF 2"() -> (w5527:dbl)
                n3979 = local read "Stroke"() -> (w5510:dbl)
                n3980 = Less?(x=w5510, y=w5504) -> (x < y?=w5507:bool)
                n3981 = In Range and Coerce(upper limit=w5508, x=w5510, lower limit=w5509) -> (In Range?=w5506:bool)  [unwired: 1 out]
                n3982 = Absolute Value(x=w5532) -> (abs(x)=w5530:dbl)
                n3983 = case shown="63.." w5524 {
                  tunnel: [2 3 3 1] -> w5517
                  frame 61, 62 {
                  }
                  frame 63.. {
                  }
                  frame ..0 {
                  }
                  frame 10..60, Default {
                  }
                }
                n3984 = case shown="True" w5518 {
                  tunnel: [1 3] -> w5516
                  frame False {
                  }
                  frame True {
                  }
                }
                n3985 = case shown="True" w5521 {
                  tunnel: [1 2] -> w5515
                  frame False {
                  }
                  frame True {
                  }
                }
                n3986 = Multiply(x=1.2 ("y"), y=0.95) -> (x*y=w5494:dbl)
                n3987 = case shown="1..10, Default" w5528 {
                  tunnel: [1 3] -> w5535
                  frame 1..10, Default {
                  }
                  frame 11.. {
                  }
                }
                n3988 = case shown="0..10, Default" w5527 {
                  tunnel: [1 2 3] -> w5534
                  frame 0..10, Default {
                  }
                  frame 11, 12 {
                  }
                  frame 13.. {
                  }
                }
                n3989 = case shown="3601.." w5530 {
                  tunnel: [1 2 3] -> w5529
                  frame 0..3000, Default {
                    # "Normal"
                  }
                  frame 3001..3600 {
                  }
                  frame 3601.. {
                  }
                }
                n3990 = Or(x=w5507, y=w5506) -> (x .or. y?=w5505:bool)
                n3991 = Greater Or Equal?(x=w5510, y=w5494) -> (x >= y?=w5497:bool)
                n3992 = case shown="0, 1, Default" w5510 {
                  tunnel: [1 3] -> w5493
                  frame 0, 1, Default {
                  }
                  frame 2.. {
                  }
                }
                n3993 = case shown="True" w5497 {
                  tunnel: [1 3] -> w5492
                  frame False {
                  }
                  frame True {
                  }
                }
                n3994 = case shown="True" w5505 {
                  tunnel: [1 2] -> w5491
                  frame False {
                  }
                  frame True {
                  }
                }
                n3995 = Build Array(w5517, w5516, w5515) -> (w5514:i32[])
                n3996 = Number To Decimal String(number=w5529) -> (decimal integer string=→"sp_st":string)  [unwired: 1 in]
                n3997 = Array Max & Min(array=w5514) -> (max value=w5511:i32)  [unwired: 3 out]
                "TEMP STATE" <- w5511
                n3998 = Number To Decimal String(number=w5535) -> (decimal integer string=w5538:string)  [unwired: 1 in]
                n3999 = Number To Decimal String(number=w5534) -> (decimal integer string=w5536:string)  [unwired: 1 in]
                n4000 = Number To Decimal String(number=w5511) -> (decimal integer string=→"temp_st":string)  [unwired: 1 in]
                n4001 = Build Array(w5493, w5492, w5491) -> (w5490:i32[])
                n4002 = local write "nl_st"(w5538) -> ()
                n4003 = local write "ff_st"(w5536) -> ()
                n4004 = Number To Decimal String(number=1) -> (decimal integer string=w5533:string)  [unwired: 1 in]
                n4005 = Array Max & Min(array=w5490) -> (max value=w5489:i32)  [unwired: 3 out]
                n4006 = local write "Air temp"(w5533) -> ()
                n4007 = Number To Decimal String(number=w5489) -> (decimal integer string=w5488:string)  [unwired: 1 in]
                n4008 = local write "Stroke Ln 2"(w5488) -> ()
              }
            }
            n4009 = local read "Stroke Ln 2"() -> (w5400:string)
            n4010 = local read "nl_st"() -> (w5406:string)
            n4011 = local read "ff_st"() -> (w5403:string)
            n4012 = local read "sp_st"() -> (w5404:string)
            n4013 = local read "temp_st"() -> (w5405:string)
            n4014 = local read "Air temp"() -> (w5399:string)
            n4015 = Replace Array Subset(array="in", new element #1=w5406, index #1=1 ("index"), new element #2=w5403, index #2=2 ("index"), new element #3=w5405, index #3=3 ("index"), new element #4=w5404, index #4=4 ("index"), new element #5=w5400, index #5=5 ("index"), new element #6=w5399, index #6=6 ("index"), new element #7="Sensor State" ("new element/subarray"), index #7=0 ("index")) -> (→"out":string[])
          }
        }
        n4016 = Wait (ms)(milliseconds to wait=u32 10) -> ()  [unwired: 1 out]
        n4017 = local read "Quit"() -> (w5394:bool)
      }
      n4018 = while {
        stop <- w5369 stop-if-true
        n4019 = local read "run replace"() -> (w5371:bool)
        n4020 = Wait (ms)(milliseconds to wait=u32 100) -> ()  [unwired: 1 out]
        n4021 = Equal?(x="FLAG 2", y=0.0) -> (x = y?=w5372:bool)
        n4022 = case shown="True" w5372 {
          frame False {
          }
          frame True {
            n4023 = local write "FLAG 2"(100.0 ("FLAG 2")) -> ()
            n4024 = call <vilib>:"Read Characters From File.vi"("file path (dialog if empty)"=path "C:/LAB-IQ-NXT/WO 2449 TT.sig", "convert eol? (no:F)"=FALSE ("append to file? (new file:F)")) -> ("character string"=w5375:string)  [unwired: 4 in, 3 out]
            n4025 = call <vilib>:"Read Characters From File.vi"("file path (dialog if empty)"=path "C:/LAB-IQ-NXT/WO 2449 TRH.sig", "convert eol? (no:F)"=FALSE ("append to file? (new file:F)")) -> ("character string"=w5376:string)  [unwired: 4 in, 3 out]
            n4026 = Decimal String To Number(string=w5375) -> (number=w5377:i32)  [unwired: 2 in, 1 out]
            n4027 = local write "Total No. of Tests"(w5377) -> ()
            n4028 = Decimal String To Number(string=w5376) -> (number=w5380:i32)  [unwired: 2 in, 1 out]
            n4029 = local write "SEN.RUN HRS"(w5380) -> ()
          }
        }
        n4030 = case shown="True" w5371 {
          frame False {
          }
          frame True {
            n4031 = Equal?(x="FLAG 4", y=0.0) -> (x = y?=w5384:bool)
            n4032 = case shown="False" w5384 {
              frame False {
                n4033 = Get Date/Time In Seconds() -> (seconds since 1Jan1904=w5390:timestamp)
                n4034 = local read "START 3"() -> (w5388:dbl)
                n4035 = To Double Precision Float(number=w5390) -> (double precision float=w5389:dbl)
                n4036 = Subtract(x=w5389, y=w5388) -> (x-y=→"SENSOR TIME":dbl)
              }
              frame True {
                n4037 = Get Date/Time In Seconds() -> (seconds since 1Jan1904=w5392:timestamp)
                n4038 = local write "FLAG 4"(100.0 ("FLAG")) -> ()
                n4039 = To Double Precision Float(number=w5392) -> (double precision float=→"START 3":dbl)
              }
            }
          }
        }
        n4040 = local read "Quit"() -> (w5369:bool)
      }
      n4041 = while {
        shift-right: [w5169] -> _
        shift-left: _ -> [w5170]
        tunnel: [w5165] -> _
        i -> [w5165]
        stop <- w5164 stop-if-true
        n4042 = Wait (ms)(milliseconds to wait=u32 50 ("Refresh Rate (ms)")) -> ()  [unwired: 1 out]
        n4043 = local read "Json End Flg"() -> (w5166:bool)
        n4044 = Not(x="Upld AR 2") -> ()  [unwired: 1 out]
        n4045 = local read "Upld AR 2"() -> (w5167:bool)
        n4046 = call "Elapsed Time9"("Time Target (s)"="Sen.Upload Rate (s)", "Reset"=FALSE, "Auto Reset"=TRUE) -> ("Time has Elapsed"=w5176:bool)  [unwired: 9 in, 7 out]
        n4047 = Or(x=w5176, y=w5166) -> (x .or. y?=w5172:bool)
        n4048 = case shown="True" w5172 {
          frame False {
          }
          frame True {
            w5268 = "\"SensorName\":\"" ("string")
            w5238 = " \"},{"
            w5263 = "\",\"SensorState\":\""
            w5265 = "\",\"SensorModelNumber\":\"" ("string")
            w5264 = "\",\"SensorRuntimeHours\":\"" ("string")
            n4049 = local read "model num"() -> (w5262:string[])
            n4050 = local read "Sensor name"() -> (w5281:string[])
            n4051 = local read "run"() -> (w5252:string[])
            n4052 = local read "SENSOR TIME"() -> (w5208:dbl)
            n4053 = local read "out"() -> (w5201:string[])
            n4054 = local read "Total No. of Tests"() -> (w5206:dbl)
            n4055 = Select(t=60.0, s="Run test 3", f=3600.0) -> (s? t:f=w5216:dbl)
            n4056 = Index Array(array=w5262, index #1=1 ("index")) -> (element #1=w5261:string, element #2=w5260:string, element #3=w5259:string, element #4=w5258:string, element #5=w5257:string, element #6=w5256:string)  [unwired: 5 in]
            n4057 = Index Array(array=w5252, index #1=1 ("index")) -> (element #1=w5251:string, element #2=w5250:string, element #3=w5249:string, element #4=w5248:string, element #5=w5247:string, element #6=w5246:string)  [unwired: 5 in]
            n4058 = Index Array(array=w5281, index #1=1 ("index")) -> (element #1=w5280:string, element #2=w5279:string, element #3=w5278:string, element #4=w5277:string, element #5=w5267:string, element #6=w5266:string)  [unwired: 5 in]
            n4059 = Index Array(array=w5201, index #1=1 ("index")) -> (element #1=w5233:string, element #2=w5232:string, element #3=w5231:string, element #4=w5230:string, element #5=w5229:string, element #6=w5228:string)  [unwired: 5 in]
            n4060 = local read "SEN.RUN HRS"() -> (w5204:dbl)
            n4061 = Divide(x=w5208, y=w5216) -> (x/y=w5215:dbl)
            n4062 = Increment(x=w5215) -> (x+1=w5211:dbl)
            n4063 = Number To Decimal String(number=w5211) -> (decimal integer string=→"run hrs":string)  [unwired: 1 in]
            n4064 = Divide(x=w5204, y=3600.0 ("f")) -> (x/y=w5199:dbl)
            n4065 = Round To Nearest(number=w5199) -> (nearest integer value=w5197:dbl)
            n4066 = Number To Decimal String(number=w5197) -> (decimal integer string=w5198:string)  [unwired: 1 in]
            n4067 = Number To Decimal String(number=w5206) -> (decimal integer string=w5207:string)  [unwired: 1 in]
            n4068 = local read "Model No"() -> (w5212:string)
            n4069 = local read "UUID"() -> (w5307:string)
            n4070 = local read "Serial No"() -> (w5311:string)
            n4071 = local read "Secret Key"() -> (w5312:string)
            n4072 = Concatenate Strings("\",\"MachineSerialNumber\":\"" ("string"), w5311) -> (w5315:string)
            n4073 = Concatenate Strings("\",\"ModelNumber\":\"" ("string"), w5212) -> (w5213:string)
            n4074 = Concatenate Strings("\",\"MachineRuntimeHours\":\"" ("string"), w5198) -> (w5316:string)
            n4075 = Concatenate Strings("\",\"MachineRuntimeCycles\":\"", w5207) -> (w5309:string)
            n4076 = Concatenate Strings(w5265, w5261) -> (w5295:string)
            n4077 = Concatenate Strings(w5264, w5251) -> (w5296:string)
            n4078 = Concatenate Strings(w5263, w5233) -> (w5294:string)
            n4079 = Concatenate Strings(w5315, w5213, w5316, w5309) -> (w5318:string)
            n4080 = Concatenate Strings(w5265, w5260) -> (w5292:string)
            n4081 = Concatenate Strings(w5264, w5250) -> (w5291:string)
            n4082 = Concatenate Strings(w5263, w5232) -> (w5293:string)
            n4083 = Concatenate Strings(w5265, w5259) -> (w5287:string)
            n4084 = Concatenate Strings(w5264, w5249) -> (w5288:string)
            n4085 = Concatenate Strings(w5263, w5231) -> (w5286:string)
            n4086 = Concatenate Strings(w5265, w5258) -> (w5284:string)
            n4087 = Concatenate Strings(w5264, w5248) -> (w5283:string)
            n4088 = Concatenate Strings(w5263, w5230) -> (w5285:string)
            n4089 = Concatenate Strings(w5295, w5296, w5294) -> (w5297:string)
            n4090 = Concatenate Strings(w5265, w5257) -> (w5274:string)
            n4091 = Concatenate Strings(w5264, w5247) -> (w5275:string)
            n4092 = Concatenate Strings(w5265, w5256) -> (w5271:string)
            n4093 = Concatenate Strings(w5264, w5246) -> (w5270:string)
            n4094 = Concatenate Strings(w5263, w5229) -> (w5273:string)
            n4095 = Concatenate Strings(w5263, w5228) -> (w5272:string)
            n4096 = Concatenate Strings("{\"SecretKey\":\"", w5312, w5318, "\",\"UUID\" : \"", w5307, "\",\"SensorInformation\":", "[{" ("string")) -> (w5245:string)
            n4097 = Concatenate Strings(w5292, w5291, w5293) -> (w5290:string)
            n4098 = Concatenate Strings(w5287, w5288, w5286) -> (w5289:string)
            n4099 = Concatenate Strings(w5284, w5283, w5285) -> (w5282:string)
            n4100 = Concatenate Strings(w5274, w5275, w5273) -> (w5276:string)
            n4101 = Concatenate Strings(w5271, w5270, w5272) -> (w5269:string)
            n4102 = Concatenate Strings(w5268, w5280, w5297, w5238) -> (w5244:string)
            n4103 = Concatenate Strings(w5268, w5279, w5290, w5238) -> (w5243:string)
            n4104 = Concatenate Strings(w5268, w5278, w5289, w5238) -> (w5242:string)
            n4105 = Concatenate Strings(w5268, w5277, w5282, w5238) -> (w5241:string)
            n4106 = Concatenate Strings(w5268, w5267, w5276, w5238) -> (w5240:string)
            n4107 = Concatenate Strings(w5268, w5266, w5269, "\"}" ("string")) -> (w5239:string)
            n4108 = Concatenate Strings(w5245, w5244, w5243, w5242, w5241, w5240, w5239, "]}" ("string")) -> (w5236:string)
            n4109 = local read "SEN.RUN HRS"() -> (w5203:dbl)
            n4110 = disable-structure shown="Disabled" {
              frame Disabled {
                n4111 = local read "state"() -> (w5322:string[])
                n4112 = Delete From Array(array=w5322, index=0) -> (array with subset deleted=w5320:string[])  [unwired: 1 in, 1 out]
                n4113 = for {
                  N: 6 -> [_]
                  tunnel: w5320 -> [w5333] mode=indexing
                  tunnel: [w5332] -> w5319 mode=indexing
                  n4114 = Equal?(x=w5333, y="Warning") -> (x = y?=w5329:bool)
                  n4115 = Equal?(x=w5333, y="Healthy") -> (x = y?=w5326:bool)
                  n4116 = Select(t="2" ("y"), s=w5329, f="3" ("y")) -> (s? t:f=w5324:string)
                  n4117 = Select(t="1" ("y"), s=w5326, f=w5324) -> (s? t:f=w5332:string)
                }
                "state1" <- w5319
              }
              frame Enabled {
              }
            }
            n4118 = stacked-sequence {
              tunnel: w5236 -> [w5344 _ _]
              tunnel: [_ _ w5360] -> _
              frame #0 {
                (unwired) FALSE ("convert eol (F)")
                w5346 = enum16{"start", "end", "current"}."start" ("pos mode (0:2)")
                n4119 = local read "Path"() -> (w5340:path)
                n4120 = Path To String(path=w5340) -> (string=w5352:string)
                n4121 = Concatenate Strings(w5352, "\\", "Sensor File Name") -> (w5353:string)
                n4122 = local write "standard output 2"(" ") -> ()
                n4123 = String To Path(string=w5353) -> (path=w5343:path)
                n4124 = call <vilib>:"Open_Create_Replace File.vi"("advisory dialog? (display:T)"=FALSE, "function (open:0)"=T28."create or replace", "file path"=w5343) -> ("error out"=w5356:errorcluster, "refnum"=w5355:refnum<file>)  [unwired: 5 in, 2 out]
                n4125 = Set File Position(refnum=w5355, from (0:start)=w5346, error in=w5356) -> (refnum out=w5336:refnum<file>, error out=w5335:errorcluster)  [unwired: 1 in]
                n4126 = Write to Binary File(file (use dialog)=w5336, data=" ", error in=w5335, 5:FALSE ("prepend array or string size? (T)")) -> (refnum out=w5347:refnum<file>, error out=w5348:errorcluster)  [unwired: 2 in, 1 out]
                n4127 = Set File Position(offset (in bytes) (0)=w5346, refnum=w5347, error in=w5348) -> (refnum out=w5339:refnum<file>, error out=w5338:errorcluster)  [unwired: 1 in]
                n4128 = Write to Binary File(file (use dialog)=w5339, data=w5344, error in=w5338, 5:FALSE ("prepend array or string size? (T)")) -> (error out=w5342:errorcluster)  [unwired: 2 in, 2 out]
                n4129 = flat-sequence {
                  tunnel: w5343 -> [w5358]
                  tunnel: w5342 -> [_]
                  frame #0 {
                    n4130 = call <vilib>:"Read Characters From File.vi"("file path (dialog if empty)"=w5358) -> ("character string"=→"Sensor Health JSON string":string)  [unwired: 5 in, 3 out]
                  }
                }
                "SinglePoint  2" <- w5344
              }
              frame #1 {
              }
              frame #2 {
                (unwired) "\"Stored\": true" ("string")
                n4131 = call <vilib>:"System Exec.vi"("run minimized? (F)"=TRUE, "wait until completion? (T)"=TRUE, "working directory"=path "C:/LAB-IQ-NXT", "command line"="C:\\LAB-IQ-NXT\\JPostH.bat") -> ("standard error"=→"Respose From Server 2":string, "standard output"=w5363:string)  [unwired: 4 in, 2 out]
                "standard output 2" <- w5363
                n4132 = Match Pattern(string=w5363, regular expression="JSONH Check String") -> (match substring=w5361:string, offset past match=w5360:i32)  [unwired: 1 in, 2 out]
                n4133 = Equal?(x=w5361, y="JSONH Check String") -> (x = y?=→"Upload \nConfirmed 2":bool)
              }
            }
            n4134 = Divide(x=w5203, y=3600.0 ("f")) -> (x/y=w5196:dbl)
            n4135 = local read "run time"() -> (w5253:string[])
            n4136 = Round To Nearest(number=w5196) -> (nearest integer value=w5195:dbl)
            n4137 = Number To Decimal String(number=w5195) -> (decimal integer string=w5194:string)  [unwired: 1 in]
            n4138 = Index Array(array="Sensor Information", index (col) #1=0 ("disabled index (col)"), index (col) #2=1 ("index (col)"), index (col) #3=2 ("index (col)"), index (col) #4=3 ("index (col)")) -> (element #1=→"Sensor name":string[], element #2=→"model num":string[], element #3=→"run time":string[], element #4=→"state":string[])  [unwired: 4 in]
            n4139 = Insert Into Array(array=w5253, index=1, new element #1=w5194, new element #2=w5194, new element #3=w5194, new element #4=w5194, new element #5=w5194, new element #6=w5194) -> (w5218:string[])
            "run" <- w5218
            n4140 = local read "out"() -> (w5200:string[])
            n4141 = local read "Sensor Information"() -> (w5220:string[][])
            n4142 = Replace Array Subset(array=w5220, new element #1=w5218, index (col) #1=2 ("disabled index (col)"), new element #2=w5200, index (col) #2=3 ("index (col)")) -> (w5219:string[][])  [unwired: 2 in]
            n4143 = local write "Sensor Information"(w5219) -> ()
          }
        }
        n4144 = case shown="True" w5167 {
          frame False {
          }
          frame True {
            n4145 = Equal?(x="FLAG", y=0.0) -> (x = y?=w5184:bool)
            n4146 = case shown="False" w5184 {
              frame False {
                n4147 = Get Date/Time In Seconds() -> (seconds since 1Jan1904=w5190:timestamp)
                n4148 = local read "START 2"() -> (w5188:dbl)
                n4149 = To Double Precision Float(number=w5190) -> (double precision float=w5189:dbl)
                n4150 = Subtract(x=w5189, y=w5188) -> (x-y=→"SENSOR TIME  2":dbl)
              }
              frame True {
                n4151 = Get Date/Time In Seconds() -> (seconds since 1Jan1904=w5192:timestamp)
                n4152 = To Double Precision Float(number=w5192) -> (double precision float=→"START 2":dbl)
                n4153 = local write "FLAG"(100.0 ("FLAG")) -> ()
              }
            }
          }
        }
        n4154 = disable-structure shown="Disabled" {
          disable-tunnel: w5170 -> [w5179 _]
          disable-tunnel: [w5178 _] -> w5169
          frame Disabled {
            n4155 = local read "Json St Flg"() -> (w5177:bool)
            n4156 = case shown="True" w5177 {
              tunnel: w5179 -> [w5180 w5182]
              tunnel: [w5180 w5181] -> w5178
              frame False {
              }
              frame True {
                n4157 = Increment(x=w5182) -> (x+1=w5181:dbl)
                "T cycle" <- w5181
                n4158 = local write "Json St Flg"(FALSE ("Json St Flg")) -> ()
              }
            }
          }
          frame Enabled {
          }
        }
        n4159 = local read "Quit"() -> (w5164:bool)
      }
    }
    frame Enabled {
